vi "Calculate Blood Pressure.vi"(8 "error in (no error)":errorcluster, 9 "Peak Amplitudes":dbl[](array[numeric]), 10 "Peak Pressures":dbl[](array[numeric]), 11 "Heart Rates":dbl[](array[numeric])) -> (0 "error out":errorcluster, 2 "Diastolic":dbl, 3 "Systolic":dbl, 4 "Output":cluster{"Pressure":dbl[], "Amplitude":dbl[]}, 5 "mean":dbl)   [LabVIEW 2017]
doc: "Description: This function shall compute the mean heart rate, systolic pressure and diastolic pressure based upon the specified inputs:\n- Heart Rates: Array of doubles representing the number of beats per minute over the period of time the measurements were acquired\n- Peak Pressures: Array of double representing peak pressures representing the amount of pressure at the peak of the measurement for each heart beat over the period of time the measurements were acquired\n- Peak Amplitudes: Array of corresponding amplitudes of the pressures, which is the value relative to the absolute minimum pressure during the period between an individual heart beat.\nThe algorithm for this function will filter outliers beyond a certain range, and compute the diastolic and systolic pressure by identifying the amplitude of the largest peak."
uses:
  <vilib>/Analysis/baseanly.llb/Mean (DBL).vi
  <vilib>/Analysis/NI_AALBase.lvlib
panel:
  # "Inputs"
  # "Outputs"
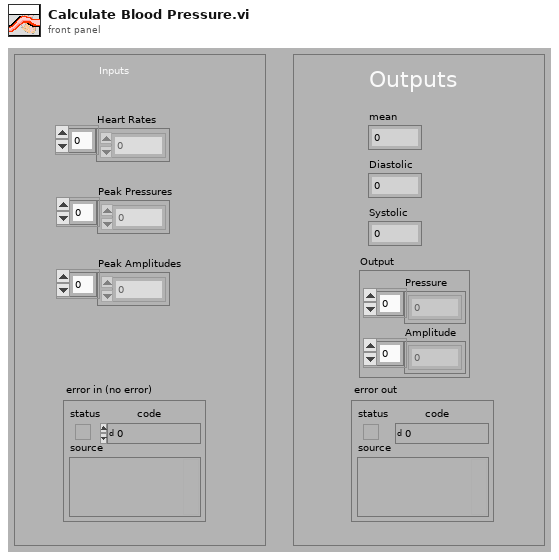
[diagram p1: front panel]
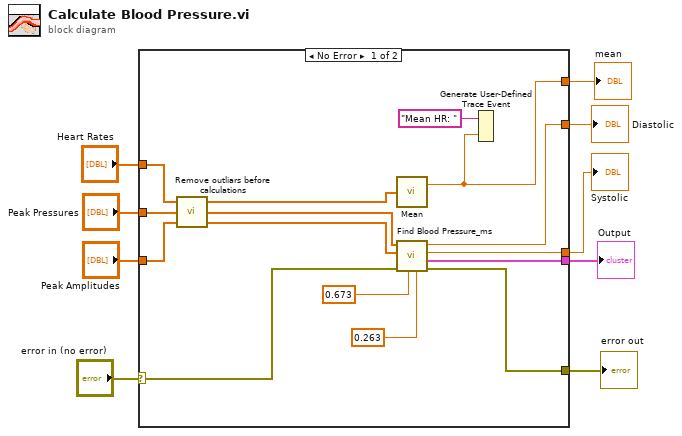
[diagram p0: block diagram]
diagram:
  n1 = case shown="No Error" "error in (no error)" {
    selector: "error in (no error)" -> [w12 w25]
    tunnel: [w24 _] -> w9
    tunnel: "Heart Rates" -> [w20 _]
    tunnel: "Peak Pressures" -> [w19 _]
    tunnel: "Peak Amplitudes" -> [w18 _]
    tunnel: [w17 _] -> w5
    tunnel: [w16 w25] -> w4
    tunnel: [w15 _] -> w3
    tunnel: [w10 _] -> w2
    frame No Error {
      n2 = call "Remove outliars before calculations.vi"("Pressure IN"=w18, "Peak Pressure IN"=w19, "Pulse Rate IN"=w20) -> ("Pressure OUT"=w23:dbl[], "Peak Pressure OUT"=w22:dbl[], "Pulse Rate OUT"=w21:dbl[])
      n3 = call-poly <vilib>:"Mean.vi"("X"=w21) -> ("mean"=w10:dbl)  [unwired: 1 out]
      n4 = call "Find Blood Pressure_ms.vi"("Systolic Threshold"=0.263, "Diastolic Threshold"=0.673, "error in (no error)"=w12, "Peak Amplitudes"=w23, "Peak Pressures"=w22) -> ("error Out"=w16:errorcluster, "Results"=w15:cluster{"Pressure":dbl[], "Amplitude":dbl[]}, "Systolic"=w17:dbl, "Diastolic"=w24:dbl)  [unwired: 3 out]
      n5 = Generate User-Defined Trace Event(1:w10, 2:"Mean HR: " ("trace string")) -> ()
    }
    frame Error {
    }
  }
  "Systolic" <- w5
  "Diastolic" <- w9
  "Output" <- w3
  "error out" <- w4
  "mean" <- w2
